vi "JRA_PID.vi"(6 "PID Out Max":dbl=1.0, 7 "Integral Reset Range":dbl=0.01, 9 "Feedback":dbl, 10 "Setpoint":dbl) -> (2 "Error":dbl, 3 "Motor Output":dbl)   [LabVIEW 2011]
panel:
  out "In Range?":bool=TRUE
  in  "input cluster":T1
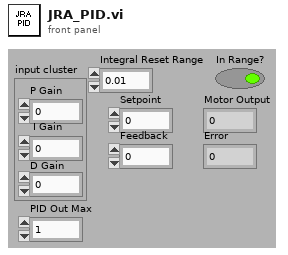
[diagram p1: front panel]
types:
  T1 = cluster{"P Gain":dbl, "I Gain":dbl, "D Gain":dbl}
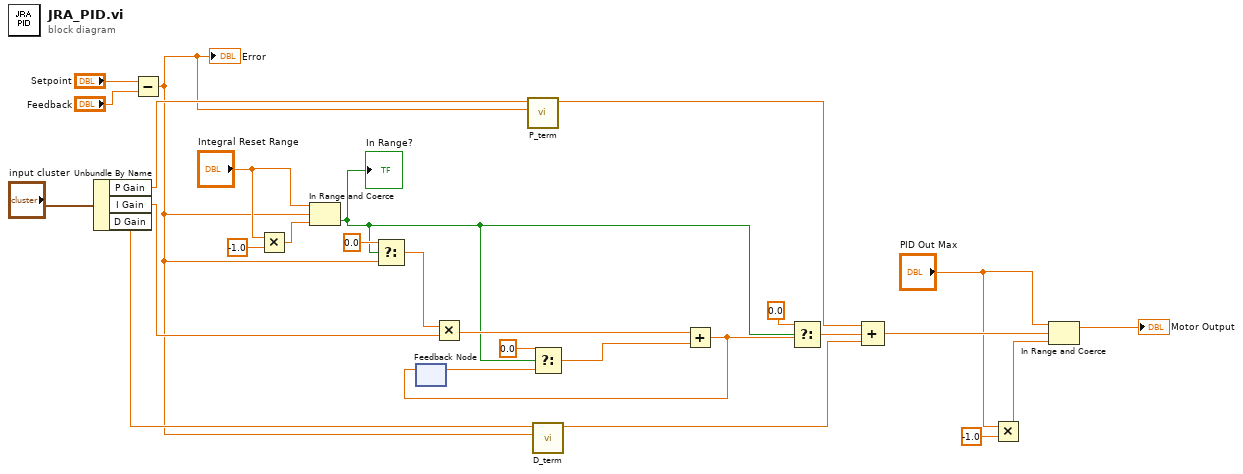
[diagram p0: block diagram]
diagram:
  n1 = Unbundle By Name("input cluster") -> ("P Gain"=w2:dbl, "I Gain"=w21:dbl, "D Gain"=w5:dbl)
  n2 = Subtract(x="Setpoint", y="Feedback") -> (x-y=w1:dbl)
  "Error" <- w1
  n3 = Multiply(x="Integral Reset Range", y=-1.0) -> (x*y=w14:dbl)
  n4 = In Range and Coerce(upper limit="Integral Reset Range", x=w1, lower limit=w14) -> (In Range?=w11:bool)  [unwired: 1 out]
  "In Range?" <- w11
  n5 = Select(t=0.0, s=w11, f=w1) -> (s? t:f=w10:dbl)
  n6 = feedback #1() -> (w16:dbl)  [unwired: 1 out]
  n7 = Multiply(x=w10, y=w21) -> (x*y=w20:dbl)
  n8 = call "P_term.vi"("Error"=w1, "P Term Gain"=w2) -> ("P Term"=w3:dbl)  [unwired: 9 out]
  n9 = Select(t=0.0, s=w11, f=w16) -> (s? t:f=w18:dbl)
  n10 = call "D_term.vi"("Error"=w1, "D Term Gain"=w5) -> ("D Term"=w4:dbl)  [unwired: 1 in, 8 out]
  n11 = Add(x=w20, y=w18) -> (x+y=w17:dbl)
  n12 = feedback-in #1(w17) -> ()
  n13 = Select(t=0.0, s=w11, f=w17) -> (s? t:f=w24:dbl)
  n14 = Compound Arithmetic op=ADD(w3, w24, w4) -> (w25:dbl)
  n15 = Multiply(x="PID Out Max", y=-1.0) -> (x*y=w7:dbl)
  n16 = In Range and Coerce(upper limit="PID Out Max", x=w25, lower limit=w7) -> (coerced(x)=→"Motor Output":dbl)  [unwired: 1 out]
